vi "SHT40_Stream_read.vi"(8 "error in (no error)":errorcluster, 11 "VISA Sesssion In":refnum<visa-resource-name>="ASRL6::INSTR") -> (0 "error out":errorcluster, 2 "output array":string[](array[string]), 3 "VISA Sesssion Out":refnum<visa-resource-name>)   [LabVIEW 2019]
panel:
  # "Johanthan Evans\n11/20/24\n\nIt does not open the serial port\nThe drycal streams data at its own speed,  This will see if data is available then read it, otherwise, it will hold the previous value. It expects an input that is: \"temp\",\"%humidity\""
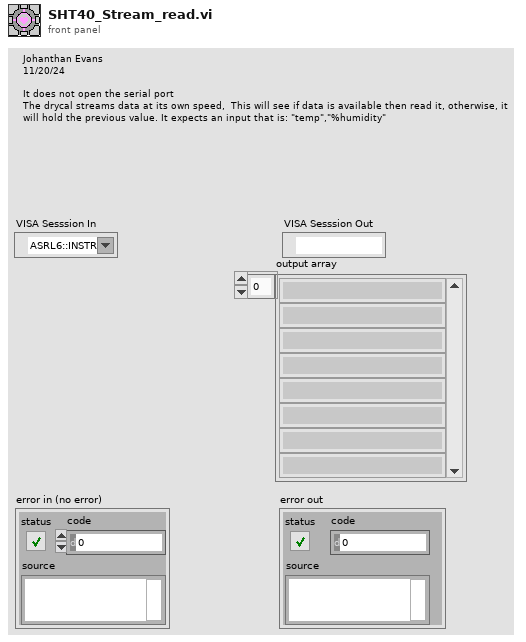
[diagram p1: front panel]
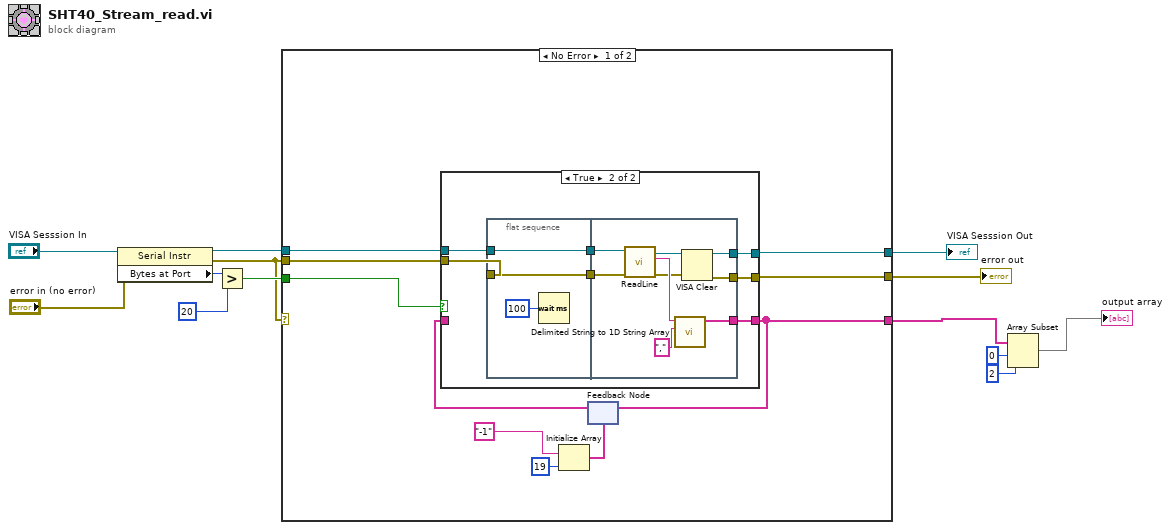
[diagram p0: block diagram]
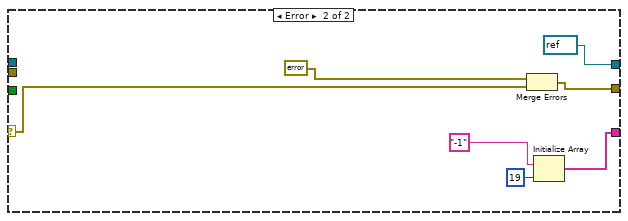
[diagram p3: hidden frame]
diagram:
  n1 = property class="Serial Instr"(reference="VISA Sesssion In", error in="error in (no error)") -> (reference out=w10:refnum<visa-resource-name>, error out=w1:errorcluster, "Bytes at Port"=w12:u32)
  n2 = Greater?(x=w12, y=u32 20) -> (0:w9:bool)
  n3 = case shown="No Error" w1 {
    selector: w1 -> [_ w51]
    tunnel: w10 -> [w23 _]
    tunnel: w1 -> [w22 _]
    tunnel: w9 -> [w21 _]
    tunnel: [w20 refnum<visa-resource-name> refnum ("VISA Sesssion Out")] -> w7
    tunnel: [w19 w50] -> w6
    tunnel: [w14 w46] -> w3
    frame No Error {
      n4 = Initialize Array("-1", 19 ("dimension size")) -> (w15:string[])
      n5 = feedback #1(w15) -> (w18:string[])
      n6 = case shown="True" w21 {
        tunnel: [w24 w33] -> w14
        tunnel: w23 -> [w25 w32]
        tunnel: w22 -> [w26 w31]
        tunnel: [w26 w28] -> w19
        tunnel: [w25 w27] -> w20
        tunnel: w18 -> [w24 _]
        frame False {
        }
        frame True {
          n7 = flat-sequence {
            tunnel: w31 -> [w35]
            tunnel: w32 -> [w36]
            tunnel: [w36] -> w30
            tunnel: [w35] -> w29
            tunnel: [w43] -> w33
            tunnel: w30 -> [w42]
            tunnel: w29 -> [w41]
            tunnel: [w38] -> w28
            tunnel: [w37] -> w27
            frame #0 {
              n8 = Wait (ms)(milliseconds to wait=u32 100) -> ()  [unwired: 1 out]
            }
            frame #1 {
              n9 = call "ReadLine.vi"("error in (no error)"=w41, "VISA Sesssion In"=w42) -> ("error out"=w39:errorcluster, "Read Line"=w45:string, "VISA Sesssion Out"=w40:refnum<visa-resource-name>)  [unwired: 7 in]
              n10 = call <vilib>:"Delimited String to 1D String Array.vi"("delimiter"=",", "delimited string"=w45) -> ("string array"=w43:string[])  [unwired: 9 in]
              n11 = VISA Clear(VISA resource name=w40, error in (no error)=w39) -> (VISA resource name out=w37:refnum<visa-resource-name>, error out=w38:errorcluster)
            }
          }
        }
      }
      n12 = feedback-in #1(w14) -> ()
    }
    frame Error {
      n13 = Merge Errors(errorcluster {"status"=TRUE, "code"=0, "source"="Process failed due to earlier errors"} ("error out"), w51) -> (w50:errorcluster)
      n14 = Initialize Array("-1", 19 ("dimension size")) -> (w46:string[])
    }
  }
  "VISA Sesssion Out" <- w7
  "error out" <- w6
  n15 = Array Subset(array=w3, index=0, length=2) -> (→"output array":string[])
